vi "ThorLabs-Connect to Scan Head.vi"(8 "error in (no error)":errorcluster) -> (0 "error out":errorcluster, 3 "ThorLabs Scan Head Connected":bool)   [LabVIEW 2020]
uses:
  LSM_SDK/ThorConfocal.lvlib
  ECU_SDK/ThorECU.lvlib
panel:
  out "DeviceCount out":i32
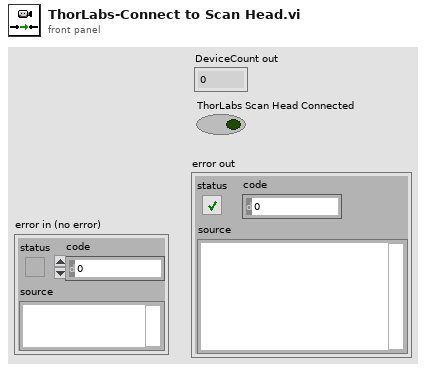
[diagram p1: front panel]
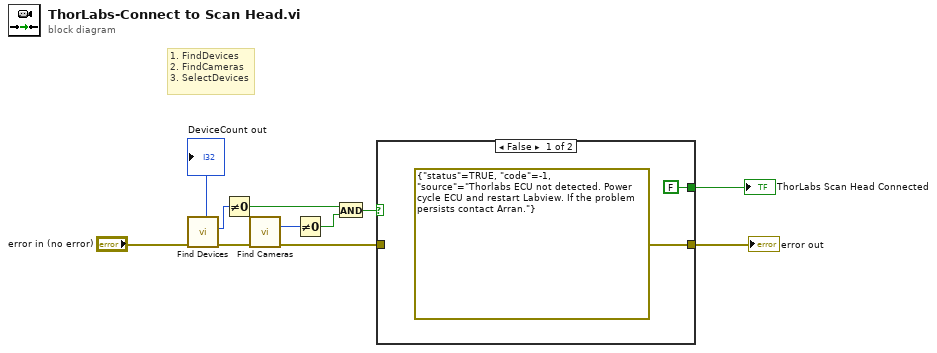
[diagram p0: block diagram]
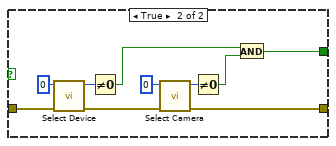
[diagram p2: hidden frame]
diagram:
  # "1. FindDevices\n2. FindCameras\n3. SelectDevices"
  n1 = call "Find Devices.vi"("error in (no error)"="error in (no error)") -> ("error out"=w11:errorcluster, "function return"=w1:i32, "DeviceCount out"=→"DeviceCount out":i32)  [unwired: 8 in]
  n2 = Not Equal To 0?(x=w1) -> (x != 0?=w6:bool)
  n3 = call "Find Cameras.vi"("error in (no error)"=w11) -> ("error out"=w7:errorcluster, "function return"=w4:i32)  [unwired: 4 in, 1 out]
  n4 = Not Equal To 0?(x=w4) -> (x != 0?=w5:bool)
  n5 = And(x=w6, y=w5) -> (x .and. y?=w10:bool)
  n6 = case shown="False" w10 {
    tunnel: w7 -> [_ w22]
    tunnel: [errorcluster {"status"=TRUE, "code"=-1, "source"="Thorlabs ECU not detected. Power cycle ECU and restart Labview. If the problem persists contact Arran."} ("error constant") w19] -> w3
    tunnel: [FALSE w14] -> w9
    frame False {
    }
    frame True {
      n7 = call "Select Device.vi"("error in (no error)"=w22, "Device"=0 ("DeviceCount")) -> ("error out"=w18:errorcluster, "function return"=w21:i32)  [unwired: 8 in]
      n8 = Not Equal To 0?(x=w21) -> (x != 0?=w16:bool)
      n9 = call "Select Camera.vi"("error in (no error)"=w18, "camera"=0) -> ("error out"=w19:errorcluster, "function return"=w17:i32)  [unwired: 4 in]
      n10 = Not Equal To 0?(x=w17) -> (x != 0?=w15:bool)
      n11 = And(x=w16, y=w15) -> (x .and. y?=w14:bool)
    }
  }
  "ThorLabs Scan Head Connected" <- w9
  "error out" <- w3
